vi "remote control.vi"   [LabVIEW 2010, in "Bluetooth.lvrbt"]
uses:
  Bluetooth.lvrbt
  <vilib>/NXT/Subs/MotorOutput.ctl
  <vilib>/NXT/Block Support/NXT_InputPort.ctl
  <vilib>/NXT/Block Support/NXT_MessageMailbox.ctl
  <vilib>/NXT/Dual Mode Library/Display/drawText.vi
  <vilib>/NXT/Dual Mode Library/Motors/ResetMotor.vi
  <vilib>/NXT/Dual Mode Library/Sensors/Touch_Pressed.vi
  <vilib>/NXT/Dual Mode Library/Motors/Rotation.vi
  <vilib>/NXT/Dual Mode Library/BT/BlueTooth_Write_Num.vi
  <vilib>/NXT/Dual Mode Library/Display/drawNumber.vi
types:
  T1 = typedef "MotorOutput.ctl" = u8
  T2 = typedef "LVHSConnector.ctl" = cluster{"Hardware":string, "Flattened String":string}
  T3 = typedef "NXT_InputPort.ctl" = u8
  T4 = typedef "NXT_MessageMailbox.ctl" = u8
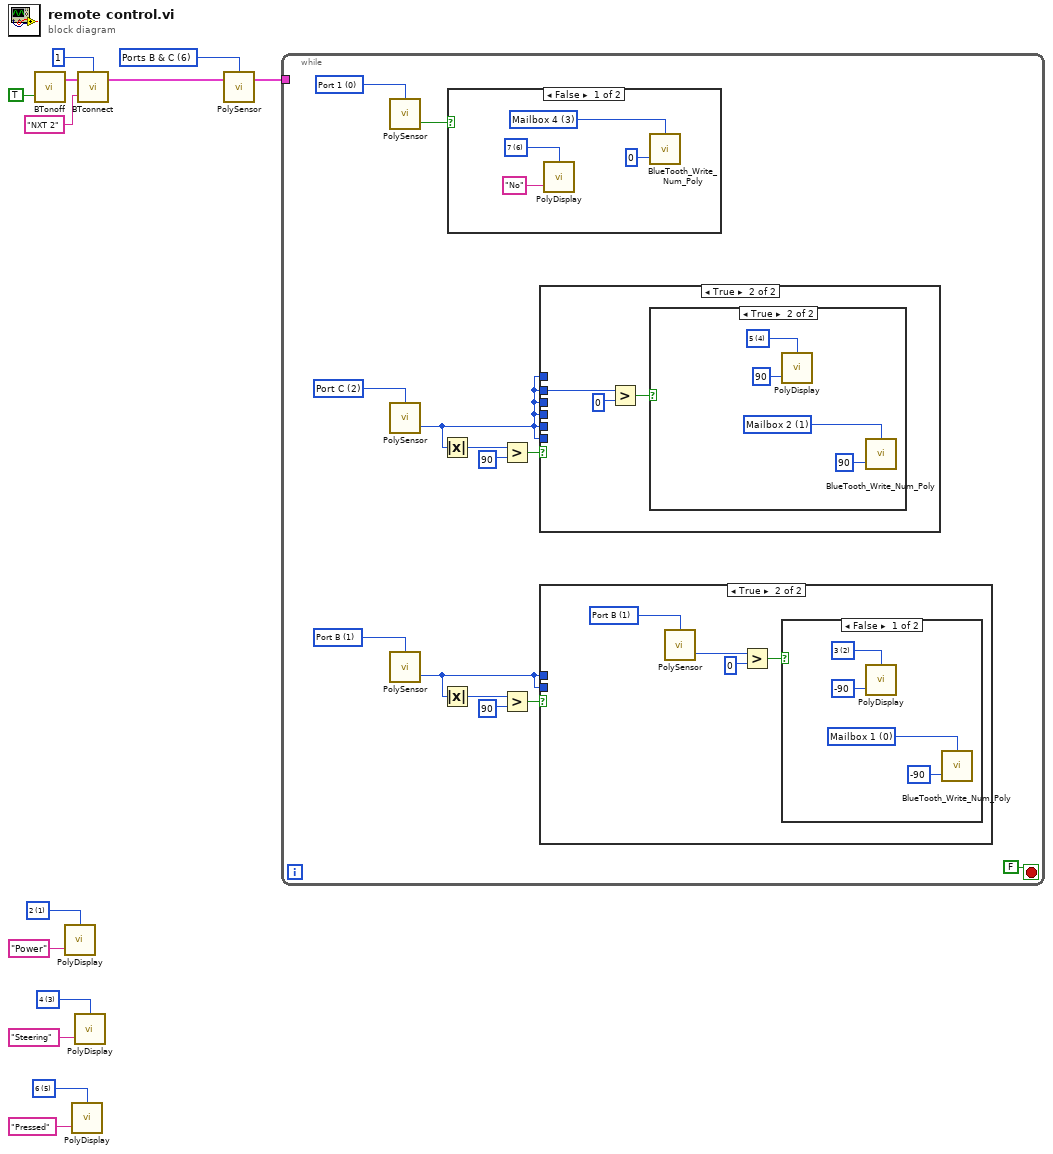
[diagram p0: block diagram]
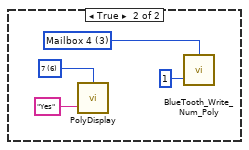
[diagram p2: hidden frame]
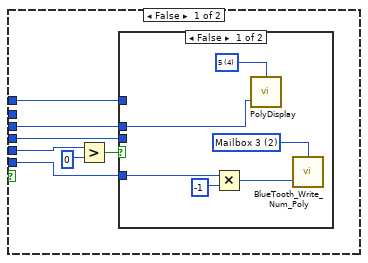
[diagram p3: hidden frame]
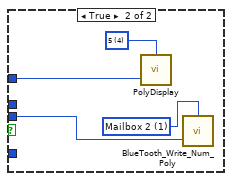
[diagram p4: hidden frame]
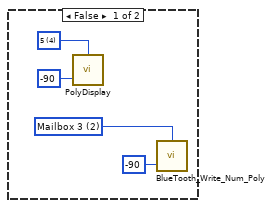
[diagram p5: hidden frame]
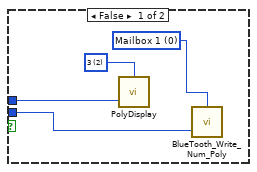
[diagram p6: hidden frame]
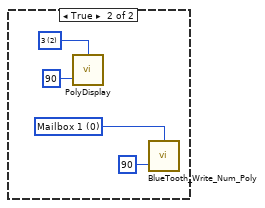
[diagram p7: hidden frame]
diagram:
  w1 = i16 5 items=["1", "2", "3", "4", "5", "6", "7", "8"] ("Line")
  w8 = i16 3 items=["1", "2", "3", "4", "5", "6", "7", "8"] ("Line")
  w10 = i16 1 items=["1", "2", "3", "4", "5", "6", "7", "8"] ("Line")
  w13 = T1 6 items=["Port A"=0, "Port B"=1, "Port C"=2, "Ports A & B"=4, "Ports A & C"=5, "Ports B & C"=6, "All Ports"=3] ("Port (All Ports)")
  n1 = call <vilib>:"BTonoff.vi"("On/Off"=TRUE) -> ("NXT"=w5:T2)  [unwired: 2 in, 1 out]
  n2 = call-poly <vilib>:"PolyDisplay.vi"("Text"="Power", "Line"=w10) -> ()  [unwired: 2 in, 1 out]
  n3 = call-poly <vilib>:"PolyDisplay.vi"("Text"="Pressed", "Line"=w1) -> ()  [unwired: 2 in, 1 out]
  n4 = call-poly <vilib>:"PolyDisplay.vi"("Text"="Steering", "Line"=w8) -> ()  [unwired: 2 in, 1 out]
  n5 = call <vilib>:"BTconnect.vi"("Partner Name"="NXT 2", "NXT"=w5, "Connection"=u8 1) -> ("NXT"=w4:T2)  [unwired: 1 out]
  n6 = call-poly <vilib>:"PolySensor.vi"("NXT"=w4, "Port (All Ports)"=w13) -> ("NXT"=w12:T2)  [unwired: 2 in]
  n7 = while {
    tunnel: w12 -> [_]
    stop <- FALSE stop-if-true
    w17 = T3 0 items=["Port 1", "Port 2", "Port 3", "Port 4"] ("Port (Port 1)")
    w24 = u8 2 items=["Port A", "Port B", "Port C"] ("Port (Port A)")
    w25 = u8 1 items=["Port A", "Port B", "Port C"] ("Port (Port A)")
    n8 = call-poly <vilib>:"PolySensor.vi"("Port (Port 1)"=w17) -> ("Yes / No"=w16:bool)  [unwired: 2 in, 1 out]
    n9 = call-poly <vilib>:"PolySensor.vi"("Port (Port A)"=w24) -> ("Angle of Rotation"=w14:i32)  [unwired: 2 in, 1 out]
    n10 = call-poly <vilib>:"PolySensor.vi"("Port (Port A)"=w25) -> ("Angle of Rotation"=w15:i32)  [unwired: 2 in, 1 out]
    n11 = Absolute Value(x=w14) -> (abs(x)=w20:i32)
    n12 = Absolute Value(x=w15) -> (abs(x)=w23:i32)
    n13 = case shown="False" w16 {
      frame False {
        w30 = i16 6 items=["1", "2", "3", "4", "5", "6", "7", "8"] ("Line")
        w28 = T4 3 items=["Mailbox 1", "Mailbox 2", "Mailbox 3", "Mailbox 4", "Mailbox 5", "Mailbox 6", "Mailbox 7", "Mailbox 8", "Mailbox 9", "Mailbox 10"] ("Mailbox")
        n14 = call-poly <vilib>:"PolyDisplay.vi"("Text"="No", "Line"=w30) -> ()  [unwired: 2 in, 1 out]
        n15 = call-poly <vilib>:"BlueTooth_Write_Num_Poly.vi"("Message"=0, "Mailbox"=w28) -> ()  [unwired: 2 in, 1 out]
      }
      frame True {
        w34 = i16 6 items=["1", "2", "3", "4", "5", "6", "7", "8"] ("Line")
        w32 = T4 3 items=["Mailbox 1", "Mailbox 2", "Mailbox 3", "Mailbox 4", "Mailbox 5", "Mailbox 6", "Mailbox 7", "Mailbox 8", "Mailbox 9", "Mailbox 10"] ("Mailbox")
        n16 = call-poly <vilib>:"PolyDisplay.vi"("Text"="Yes", "Line"=w34) -> ()  [unwired: 2 in, 1 out]
        n17 = call-poly <vilib>:"BlueTooth_Write_Num_Poly.vi"("Message"=1, "Mailbox"=w32) -> ()  [unwired: 2 in, 1 out]
      }
    }
    n18 = Greater?(x=w20, y=90) -> (0:w18:bool)
    n19 = Greater?(x=w23, y=90) -> (0:w21:bool)
    n20 = case shown="True" w18 {
      tunnel: w14 -> [w41 _]
      tunnel: w14 -> [w40 _]
      tunnel: w14 -> [_ w54]
      tunnel: w14 -> [w38 _]
      tunnel: w14 -> [w36 _]
      tunnel: w14 -> [w35 _]
      frame False {
        n21 = Greater?(x=w38, y=0) -> (0:w37:bool)
        n22 = case shown="False" w37 {
          tunnel: w41 -> [_ w49]
          tunnel: w40 -> [_ w48]
          tunnel: w36 -> [w45 _]
          tunnel: w35 -> [w42 _]
          frame False {
            w46 = i16 4 items=["1", "2", "3", "4", "5", "6", "7", "8"] ("Line")
            w47 = T4 2 items=["Mailbox 1", "Mailbox 2", "Mailbox 3", "Mailbox 4", "Mailbox 5", "Mailbox 6", "Mailbox 7", "Mailbox 8", "Mailbox 9", "Mailbox 10"] ("Mailbox")
            n23 = Multiply(x=w45, y=-1) -> (x*y=w43:i32)
            n24 = call-poly <vilib>:"PolyDisplay.vi"("number"=w42, "Line"=w46) -> ()  [unwired: 2 in, 1 out]
            n25 = call-poly <vilib>:"BlueTooth_Write_Num_Poly.vi"("Message"=w43, "Mailbox"=w47) -> ()  [unwired: 2 in, 1 out]
          }
          frame True {
            w50 = i16 4 items=["1", "2", "3", "4", "5", "6", "7", "8"] ("Line")
            w51 = T4 1 items=["Mailbox 1", "Mailbox 2", "Mailbox 3", "Mailbox 4", "Mailbox 5", "Mailbox 6", "Mailbox 7", "Mailbox 8", "Mailbox 9", "Mailbox 10"] ("Mailbox")
            n26 = call-poly <vilib>:"PolyDisplay.vi"("number"=w49, "Line"=w50) -> ()  [unwired: 2 in, 1 out]
            n27 = call-poly <vilib>:"BlueTooth_Write_Num_Poly.vi"("Message"=w48, "Mailbox"=w51) -> ()  [unwired: 2 in, 1 out]
          }
        }
      }
      frame True {
        n28 = Greater?(x=w54, y=0) -> (0:w52:bool)
        n29 = case shown="True" w52 {
          frame False {
            w55 = i16 4 items=["1", "2", "3", "4", "5", "6", "7", "8"] ("Line")
            w58 = T4 2 items=["Mailbox 1", "Mailbox 2", "Mailbox 3", "Mailbox 4", "Mailbox 5", "Mailbox 6", "Mailbox 7", "Mailbox 8", "Mailbox 9", "Mailbox 10"] ("Mailbox")
            n30 = call-poly <vilib>:"PolyDisplay.vi"("number"=-90, "Line"=w55) -> ()  [unwired: 2 in, 1 out]
            n31 = call-poly <vilib>:"BlueTooth_Write_Num_Poly.vi"("Message"=-90, "Mailbox"=w58) -> ()  [unwired: 2 in, 1 out]
          }
          frame True {
            w59 = i16 4 items=["1", "2", "3", "4", "5", "6", "7", "8"] ("Line")
            w62 = T4 1 items=["Mailbox 1", "Mailbox 2", "Mailbox 3", "Mailbox 4", "Mailbox 5", "Mailbox 6", "Mailbox 7", "Mailbox 8", "Mailbox 9", "Mailbox 10"] ("Mailbox")
            n32 = call-poly <vilib>:"PolyDisplay.vi"("number"=90, "Line"=w59) -> ()  [unwired: 2 in, 1 out]
            n33 = call-poly <vilib>:"BlueTooth_Write_Num_Poly.vi"("Message"=90, "Mailbox"=w62) -> ()  [unwired: 2 in, 1 out]
          }
        }
      }
    }
    n34 = case shown="True" w21 {
      tunnel: w15 -> [w64 _]
      tunnel: w15 -> [w63 _]
      frame False {
        w65 = i16 2 items=["1", "2", "3", "4", "5", "6", "7", "8"] ("Line")
        w66 = T4 0 items=["Mailbox 1", "Mailbox 2", "Mailbox 3", "Mailbox 4", "Mailbox 5", "Mailbox 6", "Mailbox 7", "Mailbox 8", "Mailbox 9", "Mailbox 10"] ("Mailbox")
        n35 = call-poly <vilib>:"PolyDisplay.vi"("number"=w64, "Line"=w65) -> ()  [unwired: 2 in, 1 out]
        n36 = call-poly <vilib>:"BlueTooth_Write_Num_Poly.vi"("Message"=w63, "Mailbox"=w66) -> ()  [unwired: 2 in, 1 out]
      }
      frame True {
        w69 = u8 1 items=["Port A", "Port B", "Port C"] ("Port (Port A)")
        n37 = call-poly <vilib>:"PolySensor.vi"("Port (Port A)"=w69) -> ("Angle of Rotation"=w68:i32)  [unwired: 2 in, 1 out]
        n38 = Greater?(x=w68, y=0) -> (0:w67:bool)
        n39 = case shown="False" w67 {
          frame False {
            w74 = i16 2 items=["1", "2", "3", "4", "5", "6", "7", "8"] ("Line")
            w71 = T4 0 items=["Mailbox 1", "Mailbox 2", "Mailbox 3", "Mailbox 4", "Mailbox 5", "Mailbox 6", "Mailbox 7", "Mailbox 8", "Mailbox 9", "Mailbox 10"] ("Mailbox")
            n40 = call-poly <vilib>:"PolyDisplay.vi"("number"=-90, "Line"=w74) -> ()  [unwired: 2 in, 1 out]
            n41 = call-poly <vilib>:"BlueTooth_Write_Num_Poly.vi"("Message"=-90, "Mailbox"=w71) -> ()  [unwired: 2 in, 1 out]
          }
          frame True {
            w75 = i16 2 items=["1", "2", "3", "4", "5", "6", "7", "8"] ("Line")
            w78 = T4 0 items=["Mailbox 1", "Mailbox 2", "Mailbox 3", "Mailbox 4", "Mailbox 5", "Mailbox 6", "Mailbox 7", "Mailbox 8", "Mailbox 9", "Mailbox 10"] ("Mailbox")
            n42 = call-poly <vilib>:"PolyDisplay.vi"("number"=90, "Line"=w75) -> ()  [unwired: 2 in, 1 out]
            n43 = call-poly <vilib>:"BlueTooth_Write_Num_Poly.vi"("Message"=90, "Mailbox"=w78) -> ()  [unwired: 2 in, 1 out]
          }
        }
      }
    }
  }
